vi "Mind Reading_Main.vi"() -> ()   [LabVIEW 2015]
panel:
  out "Question Number":i32
  out "Possible Results":string[](array[string])
  out "AI Question":string
  in  "Don't know":bool
  in  "No":bool
  in  "Yes":bool
  in  "Start Game":bool
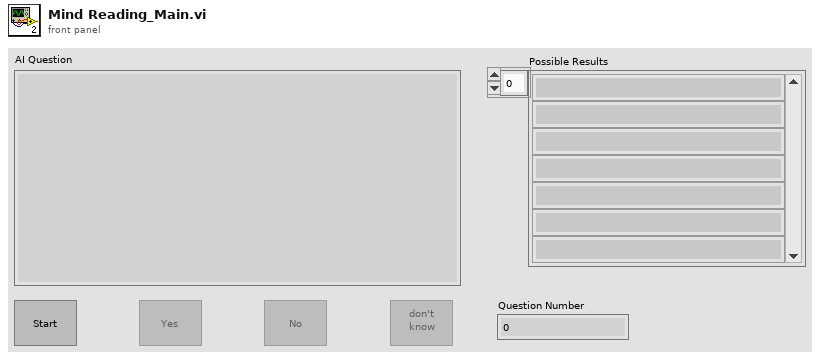
[diagram p1: front panel]
types:
  T1 = enum8{"Enabled", "Disabled", "Disabled and Grayed Out"}
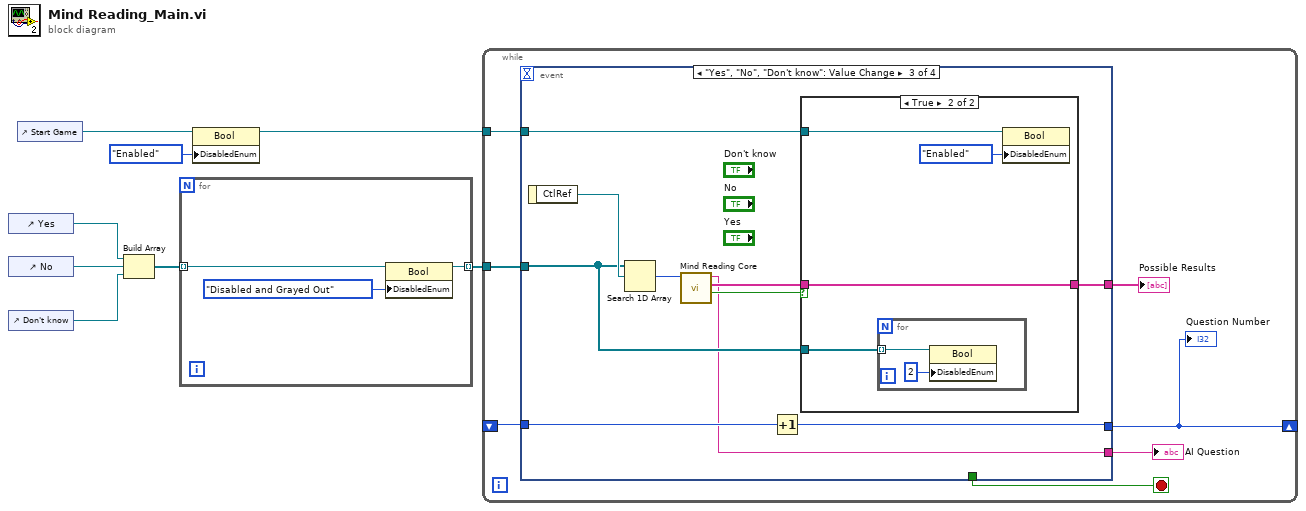
[diagram p0: block diagram]
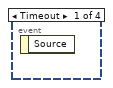
[diagram p2: hidden frame]
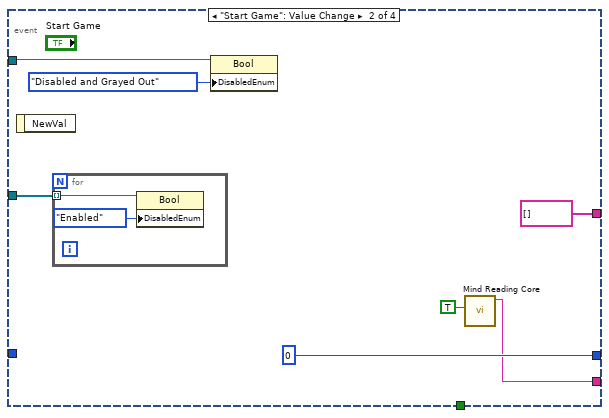
[diagram p3: hidden frame]
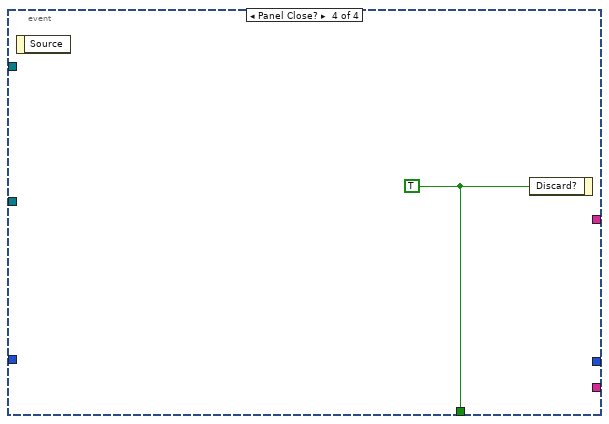
[diagram p5: hidden frame]
diagram:
  n1 = control-ref of="Yes"() -> (w8:refnum<vi>)
  n2 = control-ref of="No"() -> (w7:refnum<vi>)
  n3 = control-ref of="Don't know"() -> (w6:refnum<vi>)
  n4 = control-ref of="Start Game"() -> (w5:refnum<vi>)
  n5 = Build Array(w8, w7, w6) -> (w3:refnum<vi>[])
  n6 = for {
    tunnel: w3 -> [w11] mode=indexing
    tunnel: [w10] -> w2 mode=indexing
    n7 = property class="Bool"(reference=w11, "DisabledEnum"=T1."Disabled and Grayed Out" ("Disabled")) -> (reference out=w10:refnum<vi>)  [unwired: 1 in, 1 out]
  }
  n8 = property class="Bool"(reference=w5, "DisabledEnum"=T1."Enabled" ("Disabled")) -> (reference out=w1:refnum<vi>)  [unwired: 1 in, 1 out]
  n9 = while {
    tunnel: w2 -> [w18]
    tunnel: w1 -> [w17]
    shift-right: [w15] -> _
    shift-left: _ -> [w14]
    stop <- w16 stop-if-true
    n10 = event shown="[2] \"Yes\", \"No\", \"Don't know\": Value Change" {
      selector: _ -> [_ _ _ _]
      dyn-events: _ -> [_ _ _ _]
      timeout: _ -> [_ _ _ _]
      tunnel: w18 -> [_ w23 w31 _]
      tunnel: w17 -> [_ w25 w30 _]
      tunnel: [_ _ _ w44] -> w16
      tunnel: [_ 0 w32 _] -> w15
      tunnel: w14 -> [_ _ w33 _]
      tunnel: [_ w20 w29 _] -> w13
      tunnel: [_ string[] [] ("Possible Results") w28 _] -> w12
      event Timeout {
        n11 = event-data() -> ()  [unwired: 1 in, 1 out]
      }
      event "Start Game": Value Change {
        n12 = event-data() -> ()  [unwired: 1 in, 1 out]
        n13 = for {
          tunnel: w23 -> [w27] mode=indexing
          n14 = property class="Bool"(reference=w27, "DisabledEnum"=T1."Enabled" ("Disabled")) -> ()  [unwired: 1 in, 2 out]
        }
        n15 = property class="Bool"(reference=w25, "DisabledEnum"=T1."Disabled and Grayed Out" ("Disabled")) -> ()  [unwired: 1 in, 2 out]
        n16 = call "Mind Reading Core.vi"("FirstRun"=TRUE ("FiirstRun")) -> ("AI Question"=w20:string)  [unwired: 8 in, 2 out]
      }
      event "Yes", "No", "Don't know": Value Change {
        n17 = event-data() -> ("CtlRef"=w37:refnum<vi>)  [unwired: 1 in]
        n18 = Search 1D Array(1D array=w31, element=w37) -> (index of element=w36:i32)  [unwired: 1 in]
        n19 = call "Mind Reading Core.vi"("Answer"=w36) -> ("Results generated"=w35:bool, "Possible Results"=w34:string[], "AI Question"=w29:string)  [unwired: 8 in]
        n20 = Increment(x=w33) -> (x+1=w32:i32)
        n21 = case shown="True" w35 {
          tunnel: w34 -> [_ w38]
          tunnel: w31 -> [_ w39]
          tunnel: w30 -> [_ w41]
          tunnel: [_ w38] -> w28
          frame False {
          }
          frame True {
            n22 = for {
              tunnel: w39 -> [w43] mode=indexing
              n23 = property class="Bool"(reference=w43, "DisabledEnum"=2) -> ()  [unwired: 1 in, 2 out]
            }
            n24 = property class="Bool"(reference=w41, "DisabledEnum"=T1."Enabled" ("Disabled")) -> ()  [unwired: 1 in, 2 out]
          }
        }
      }
      event Panel Close? {
        w44 = TRUE ("Discard?")
        n25 = event-data() -> ()  [unwired: 1 in, 1 out]
        n26 = event-data("Discard?"=w44) -> ()  [unwired: 1 in, 1 out]
      }
    }
    "Question Number" <- w15
    "AI Question" <- w13
    "Possible Results" <- w12
  }
